vi "Read connection type.vi"(8 "error in (no error)":errorcluster, 11 "tcp connection in":refnum<class "tcp connection.lvclass">) -> (0 "error out":errorcluster, 2 "connection type":T1, 3 "tcp connection out":refnum<class "tcp connection.lvclass">)   [LabVIEW 2014, in "tcp connection.lvclass"]
uses:
  tcp connection.lvclass
  typedefs/connection type.ctl
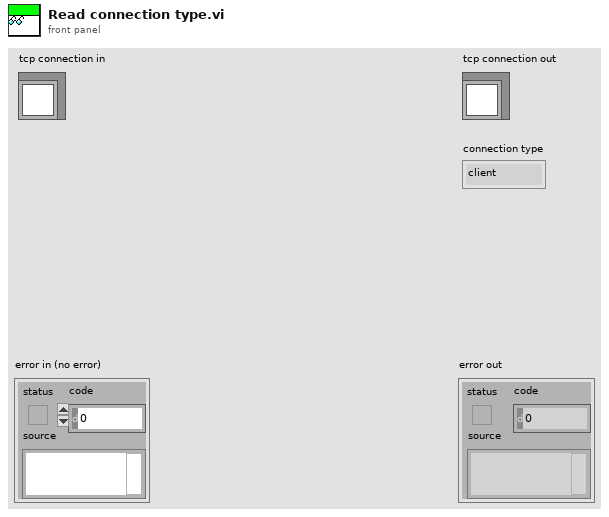
[diagram p1: front panel]
types:
  T1 = typedef "connection type.ctl" = enum16{"client", "server"}
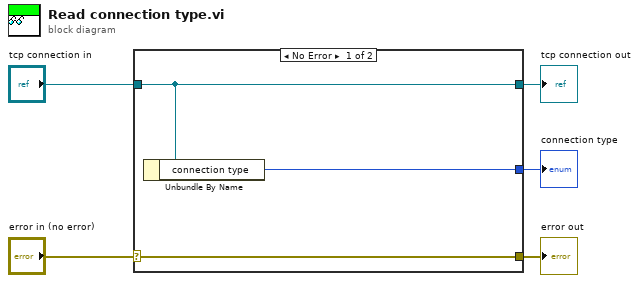
[diagram p0: block diagram]
diagram:
  n1 = case shown="No Error" "error in (no error)" {
    selector: "error in (no error)" -> [w8 w9]
    tunnel: [w8 w9] -> w4
    tunnel: [w7 w10] -> w2
    tunnel: "tcp connection in" -> [w7 w10]
    tunnel: [w6 _] -> w1
    frame No Error {
      n2 = Unbundle By Name(w7) -> ("connection type"=w6:T1)
    }
    frame Error {
    }
  }
  "error out" <- w4
  "tcp connection out" <- w2
  "connection type" <- w1
